vi "Set Value.vi"(8 "error in":errorcluster, 10 "Value":variant, 11 "MyTestHeader in":refnum<class "MyTestHeader.lvclass">) -> (0 "error out":errorcluster, 3 "MyTestHeader out":refnum<class "MyTestHeader.lvclass">)   [LabVIEW 2024, in "MyTestHeader.lvclass"]
uses:
  MyTestHeader.lvclass
  source/Cells/ColumnHeader/Column Header.lvclass
  source/Views/Cell View/Cell View.lvclass
  MyTestHeader.lvclass/MyTestHeader.ctl
  source/Color/Color.lvclass
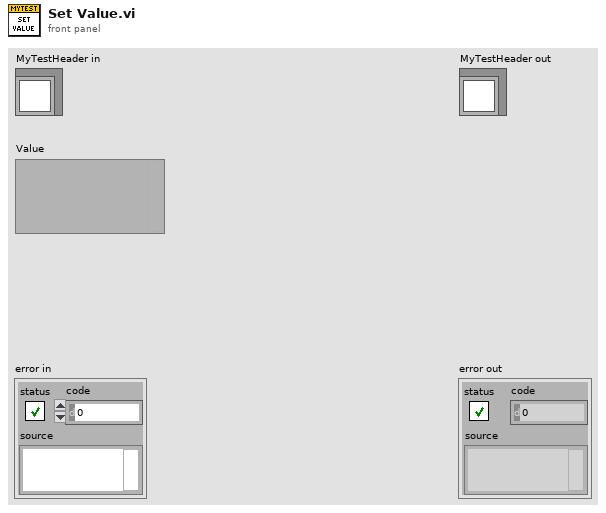
[diagram p1: front panel]
types:
  T1 = enum16{"AliceBlue", "AntiqueWhite", "Aqua", "Aquamarine", "Azure", "Beige", "Bisque", "Black", "BlanchedAlmond", "Blue", "BlueViolet", "Brown", "BurlyWood", "CadetBlue", "Chartreuse", "Chocolate", "Coral", "CornflowerBlue", "Cornsilk", "Crimson", "Cyan", "DarkBlue", "DarkCyan", "DarkGoldenrod", "DarkGray", "DarkGreen", "DarkKhaki", "DarkMagenta", "DarkOliveGreen", "DarkOrange", "DarkOrchid", "DarkRed", "DarkSalmon", "DarkSeaGreen", "DarkSlateBlue", "DarkSlateGray", "DarkTurquoise", "DarkViolet", "DeepPink", "DeepSkyBlue", "DimGray", "DodgerBlue", "Firebrick", "FloralWhite", "ForestGreen", "Fuchsia", "Gainsboro", "GhostWhite", "Gold", "Goldenrod", "Gray", "Green", "GreenYellow", "Honeydew", "HotPink", "IndianRed", "Indigo", "Ivory", "Khaki", "Lavender", "LavenderBlush", "LawnGreen", "LemonChiffon", "LightBlue", "LightCoral", "LightCyan", "LightGoldenrodYellow", "LightGray", "LightGreen", "LightPink", "LightSalmon", "LightSeaGreen", "LightSkyBlue", "LightSlateGray", "LightSteelBlue", "LightYellow", "Lime", "LimeGreen", "Linen", "Magenta", "Maroon", "MediumAquamarine", "MediumBlue", "MediumOrchid", "MediumPurple", "MediumSeaGreen", "MediumSlateBlue", "MediumSpringGreen", "MediumTurquoise", "MediumVioletRed", "MidnightBlue", "MintCream", "MistyRose", "Moccasin", "NavajoWhite", "Navy", "OldLace", "Olive", "OliveDrab", "Orange", "OrangeRed", "Orchid", "PaleGoldenrod", "PaleGreen", "PaleTurquoise", "PaleVioletRed", "PapayaWhip", "PeachPuff", "Peru", "Pink", "Plum", "PowderBlue", "Purple", "Red", "RosyBrown", "RoyalBlue", "SaddleBrown", "Salmon", "SandyBrown", "SeaGreen", "SeaShell", "Sienna", "Silver", "SkyBlue", "SlateBlue", "SlateGray", "Snow", "SpringGreen", "SteelBlue", "Tan", "Teal", "Thistle", "Tomato", "Transparent", "Turquoise", "Violet", "Wheat", "White", "WhiteSmoke", "Yellow"}
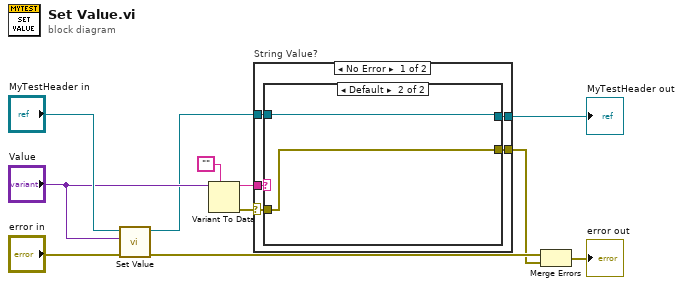
[diagram p0: block diagram]
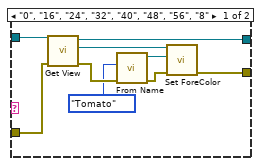
[diagram p2: hidden frame]
diagram:
  n1 = call-parent "Set Value.vi"("error in"="error in", "Value"="Value", "Cell in"="MyTestHeader in") -> ("error out"=w3:errorcluster, "Cell out"=w6:refnum<class "MyTestHeader.lvclass">)  [unwired: 7 in]
  n2 = Variant To Data(type="", Variant="Value") -> (data=w7:string, error out=w5:errorcluster)  [unwired: 1 in]
  n3 = case "String Value?" shown="No Error" w5 {
    selector: w5 -> [w14 _]
    tunnel: w7 -> [w16 _]
    tunnel: w6 -> [w15 w28]
    tunnel: [w13 w28] -> w4
    tunnel: [w12 _] -> w1
    frame No Error {
      n4 = case shown="Default" w16 {
        tunnel: w15 -> [w25 w27]
        tunnel: w14 -> [w24 w26]
        tunnel: [w22 w27] -> w13
        tunnel: [w17 w26] -> w12
        frame "0", "16", "24", "32", "40", "48", "56", "8" {
          n5 = call-dynamic "Get View.vi"("error in"=w24, "Cell in"=w25) -> ("error out"=w20:errorcluster, "View"=w23:refnum<class "Cell View.lvclass">, "Cell out"=w22:refnum<class "MyTestHeader.lvclass">)  [unwired: 7 in]
          n6 = call "From Name.vi"("error in"=w20, "Color"=T1."Tomato") -> ("error out"=w19:errorcluster, "Color out"=w21:refnum<class "Color.lvclass">)  [unwired: 8 in]
          n7 = call-dynamic "Set ForeColor.vi"("error in"=w19, "Color"=w21, "View in"=w23) -> ("error out"=w17:errorcluster)  [unwired: 7 in, 1 out]
        }
        frame Default {
        }
      }
    }
    frame Error {
    }
  }
  "MyTestHeader out" <- w4
  n8 = Merge Errors(w3, w1) -> (→"error out":errorcluster)
